vi "Sine+function.vi"(0 "Frequency (Hz)":dbl, 1 "Time (Sec)":dbl, 2 "Amplitude":dbl, 3 "DC Offset":dbl, 4 "Phase (Degrees)":dbl) -> (5 "A*sin(2*pi*f*t+phi)+B":dbl)   [LabVIEW 2010]
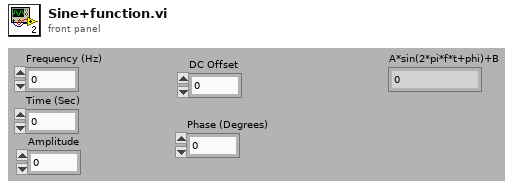
[diagram p1: front panel]
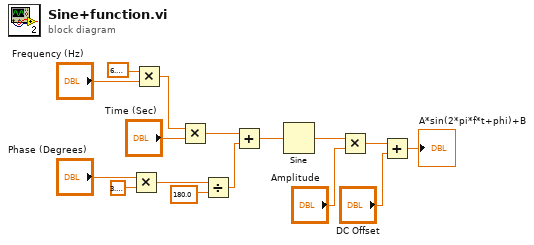
[diagram p0: block diagram]
diagram:
  n1 = Multiply(x="Phase (Degrees)", y=3.141592653589793) -> (x*y=w4:dbl)
  n2 = Multiply(x=6.283185307179586, y="Frequency (Hz)") -> (x*y=w14:dbl)
  n3 = Multiply(x=w14, y="Time (Sec)") -> (x*y=w12:dbl)
  n4 = Divide(x=w4, y=180.0) -> (x/y=w1:dbl)
  n5 = Add(x=w12, y=w1) -> (x+y=w11:dbl)
  n6 = Sine(x=w11) -> (sin(x)=w10:dbl)
  n7 = Multiply(x=w10, y="Amplitude") -> (x*y=w8:dbl)
  n8 = Add(x=w8, y="DC Offset") -> (x+y=→"A*sin(2*pi*f*t+phi)+B":dbl)
